vi "ShowMES_SFP.vi"(0 "reference in":refnum<class "Test_Base.lvclass">, 5 "error in (no error)":errorcluster) -> (14 "reference in":refnum<class "Test_Base.lvclass">, 19 "error out":errorcluster)   [LabVIEW 2022 SP3, in "Test_Base.lvlib" / "Test_Base.lvclass"]
uses:
  Test_Base.lvclass
  Components/MES_Base.lvlibp/MES_Base.lvclass
  Components/ViPER.lvlibp/ViPER.lvclass
  C:/Projects/Medulla/ViPER/Examples/Flux_Capacitor_Tester/Components/ViPER.lvlibp/ViPER.lvclass
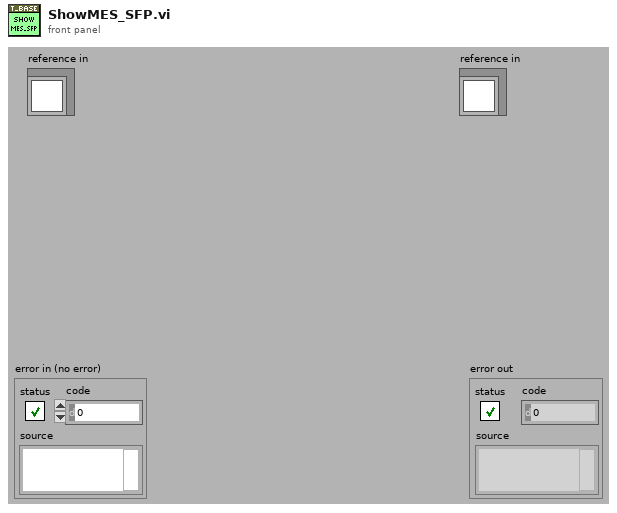
[diagram p1: front panel]
types:
  T1 = typedef "Test_Base.lvlib/Test_Base.lvclass/ObjectAttributes.ctl" = cluster{"Config":T2, "UUTIndex":i32, "Serial":string, "Batch":string, "MES":refnum<class "MES_Base.lvclass">, "TestView":refnum<class "TestView_Base.lvclass">, "LoggedIn":bool, "Abort":bool}
  T2 = typedef "Test_Base.lvlib/Test_Base.lvclass/Config.ctl" = cluster{"ContinueOnFail":bool}
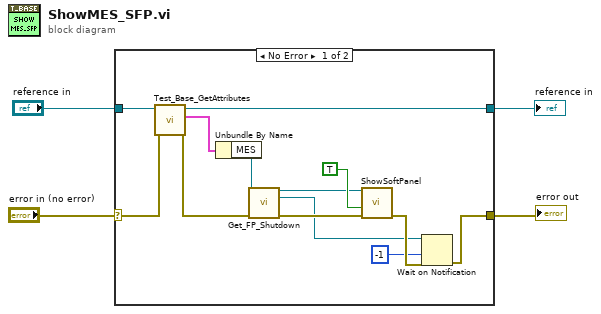
[diagram p0: block diagram]
diagram:
  n1 = case shown="No Error" "error in (no error)" {
    selector: "error in (no error)" -> [w17 w19]
    tunnel: [w7 w19] -> w3
    tunnel: [w14 w18] -> w1
    tunnel: "reference in" -> [w15 w18]
    frame No Error {
      n2 = call "Test_Base_GetAttributes.vi"("error in (no error)"=w17, "reference in"=w15) -> ("error out"=w12:errorcluster, "Data"=w16:T1, "reference out"=w14:refnum<class "Test_Base.lvclass">)  [unwired: 6 in, 1 out]
      n3 = Unbundle By Name(w16) -> ("MES"=w10:refnum<class "MES_Base.lvclass">)
      n4 = call "Get_FP_Shutdown.vi"("ViPER_Base in"=w10, "error in (no error)"=w12) -> ("ViPER_Base out"=w9:refnum<class "MES_Base.lvclass">, "SoftFP_Shutdown"=w6:refnum<notifier>, "error out"=w11:errorcluster)  [unwired: 10 in, 1 out]
      n5 = call-dynamic "ShowSoftPanel.vi"("error in (no error)"=w11, "Floating"=TRUE, "Driver in"=w9) -> ("error out"=w8:errorcluster)  [unwired: 6 in, 2 out]
      n6 = Wait on Notification(notifier=w6, timeout in ms (-1)=-1, error in (no error)=w8) -> (error out=w7:errorcluster)  [unwired: 1 in, 3 out]
    }
    frame Error {
    }
  }
  "error out" <- w3
  "reference in" <- w1
